vi "prueba5.vi"() -> ()   [LabVIEW 2011]
panel:
  out "Array":T1(array[cluster]) {"Tanque3" scale=0.0..10.0; "Tanque2" scale=0.0..10.0; "Tanque1" scale=0.0..10.0}
  # "Elaborar un programa para adicionar este cluster a un archivo de texto\nLuego deberá hacer otro programa donde lea la información del archivo \nde texto y lo coloque en el cluster."
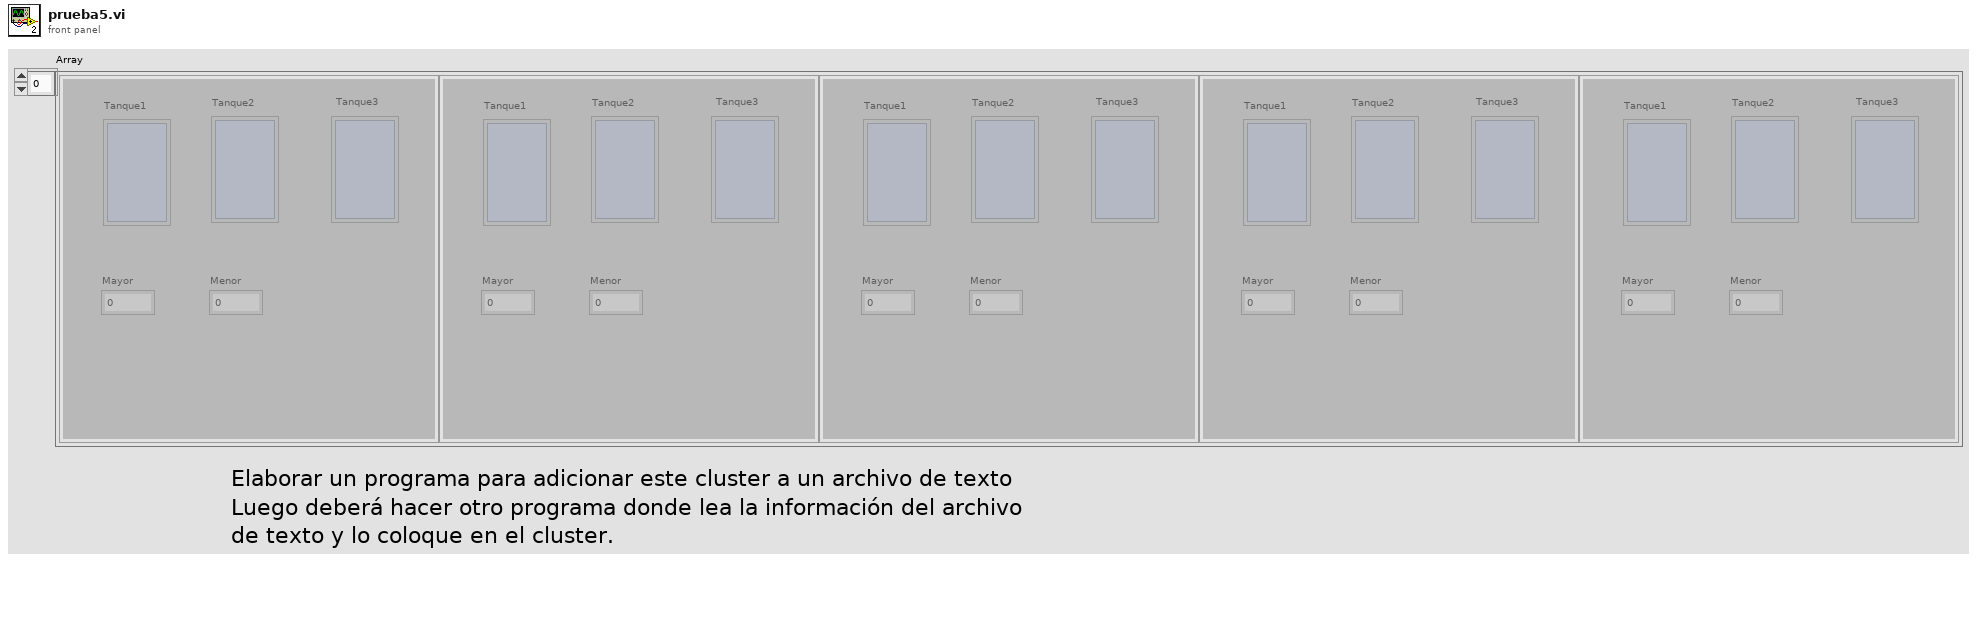
[diagram p1: front panel]
types:
  T1 = cluster{"Tanque1":dbl, "Tanque2":dbl, "Tanque3":dbl, "Mayor":dbl, "Menor":dbl}[]
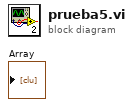
[diagram p0: block diagram]
diagram:
